vi "Single Trigger Pulse Width Upper Limit Query.vi"(8 "error in":errorcluster, 11 "Instrument Handle In":i32) -> (0 "error out":errorcluster, 2 "Upper Limit":dbl, 3 "Instrument Handle Out":i32)   [LabVIEW 8.6, in "ZTScopeM.lvlib"]
doc: "Query the upper pulse width limit."
uses:
  ZTScopeM.lvlib
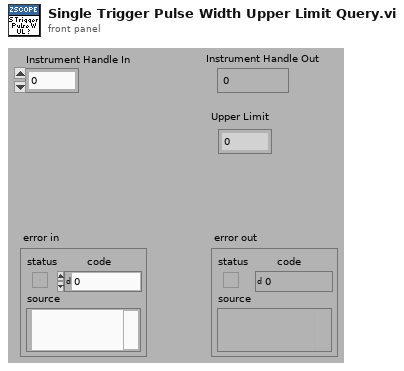
[diagram p1: front panel]
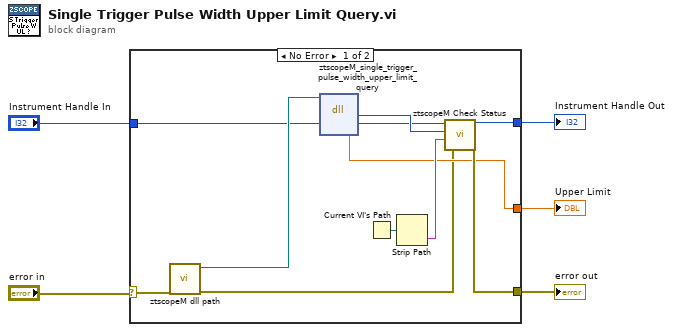
[diagram p0: block diagram]
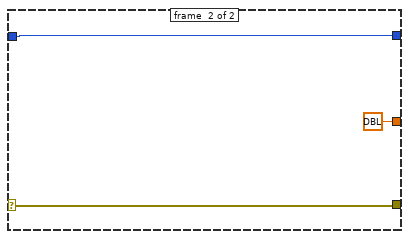
[diagram p2: hidden frame]
diagram:
  n1 = case shown="No Error" "error in" {
    selector: "error in" -> [w8 w19]
    tunnel: [w11 w19] -> w4
    tunnel: [w12 w17] -> w3
    tunnel: [w10 dbl ? ("lowerLimit")] -> w2
    tunnel: "Instrument Handle In" -> [w6 w17]
    frame #0 {
      n2 = call "ztscopeM dll path.vi"("error in (no error)"=w8) -> ("error out"=w9:errorcluster, "<instrument>.dll path"=w7:path)  [unwired: 9 in]
      n3 = dll-call lib="C:/Projects/codedepot/Teradyne/2016-1034 Teradyne ZScope API/Software/C src/ztScopeM/ZtScopeM.dll" fn="ztscopeM_single_trigger_pulse_width_upper_limit_query" ("ztscopeM.dll:ztscopeM_single_trigger_pulse_width_lower_limit_query")(path in=w7, "instrumentHandle"=w6) -> ("return type"=w16:i32, "instrumentHandle"=w15:i32, "upperLimit"=w10:dbl)  [unwired: 2 in, 3 out]
      n4 = Current VI's Path() -> (path=w14:path)
      n5 = Strip Path(path=w14) -> (name=w13:string)  [unwired: 1 out]
      n6 = call "ztscopeM Check Status.vi"("error in"=w9, "name of VI"=w13, "status (return code)"=w16, "instrument handle in"=w15) -> ("error out"=w11:errorcluster, "instrument handle out"=w12:i32)  [unwired: 2 out]
    }
    frame #1 {
    }
  }
  "Instrument Handle Out" <- w3
  "error out" <- w4
  "Upper Limit" <- w2
